vi "Core_[HSMS]Selected.vi"(8 "error in (no error)":errorcluster, 11 "HSMS Class in":refnum<class "HSMS Class.lvclass">) -> (0 "error out":errorcluster, 3 "HSMS Class out":refnum<class "HSMS Class.lvclass">)   [LabVIEW 2020, in "SECS Communication.lvlib" / "HSMS Class.lvclass"]
uses:
  HSMS Class.lvclass
  Notifier Type.ctl
  Message Packet.ctl
  Message Header.ctl
  PType.ctl
  SType.ctl
  HSMS State.ctl
  HSMS Class.lvclass/HSMS Class.ctl
  S9 Message Class/S9 Message Class.lvclass
  D:/Dropbox/SECS/SECS_GEM v1.1.2/Com/SECS Communication/SECS-II Class/SECS-II Class.lvclass
  Command Data.ctl
  SECS-II Class/SECS-II Class.lvclass
  Read Session ID.vi
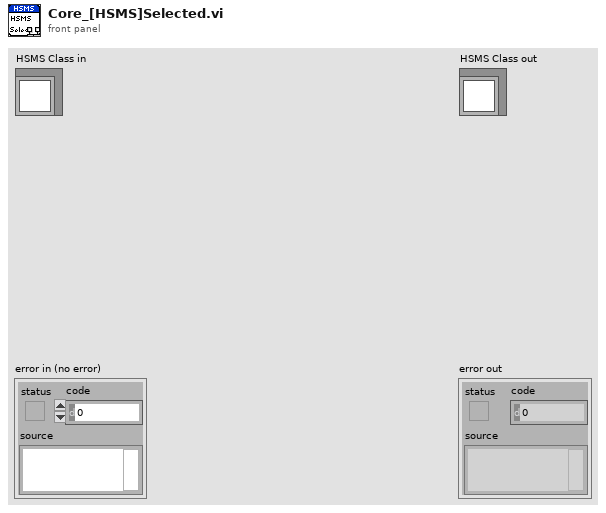
[diagram p1: front panel]
types:
  T1 = typedef "SECS Communication.lvlib/HSMS Class.lvclass/Message Packet.ctl" = cluster{"Message Header Cluster":T2, "Message Header":u8[], "Message Text":u8[]}
  T2 = typedef "SECS Communication.lvlib/HSMS Class.lvclass/Message Header.ctl" = cluster{"Byte 0-1(Session ID)":u16, "W-Bit":bool, "Byte 2":u8, "Byte 3":u8, "Byte 4(PType)":T3, "Byte 5(SType)":T4, "Byte 6-9(System Btyes)":u8[]}
  T3 = typedef "SECS Communication.lvlib/HSMS Class.lvclass/PType.ctl" = enum8{"SECS-II Encoding", "Reserved"}
  T4 = typedef "SECS Communication.lvlib/HSMS Class.lvclass/SType.ctl" = enum8{"Data Message", "Select.req", "Select.rsp", "Deselect.req", "Deselect.rsp", "Linktest.req", "Linktest.rsp", "Reject.req", "Separate.req"}
  T5 = typedef "SECS Communication.lvlib/HSMS Class.lvclass/Notifier Type.ctl" = enum16{"TCPIP Connect", "TCPIP Disconnect", "Receive Message", "Send Message", "T3 Timeout", "T6 Timeout", "T7 Timeout", "Error", "Stop"}
  T6 = typedef "SECS Communication.lvlib/HSMS Class.lvclass/HSMS State.ctl" = enum16{"[TCP/IP]Not Connect", "[HSMS]Not Selected", "[HSMS]Selected", "Stop"}
  T7 = typedef "SECS Communication.lvlib/HSMS Class.lvclass/Command Data.ctl" = cluster{"SECS-II Class":refnum<class "SECS-II Class.lvclass">, "Reply Notifier":refnum<notifier>}
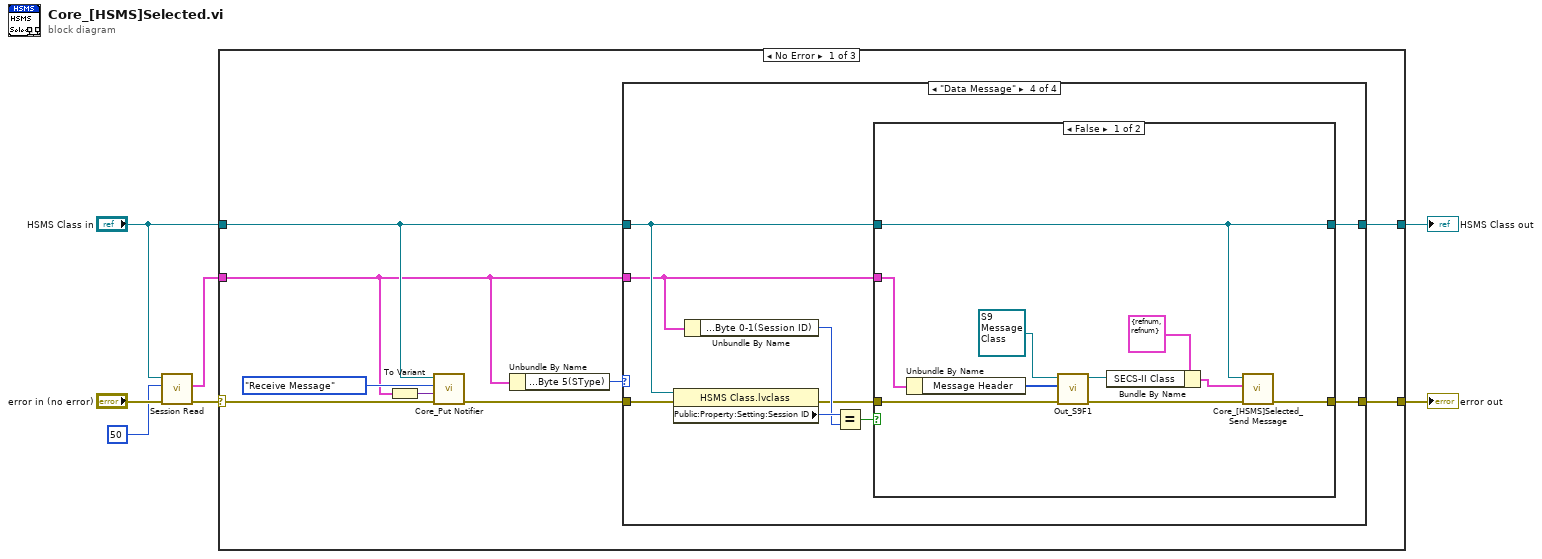
[diagram p0: block diagram]
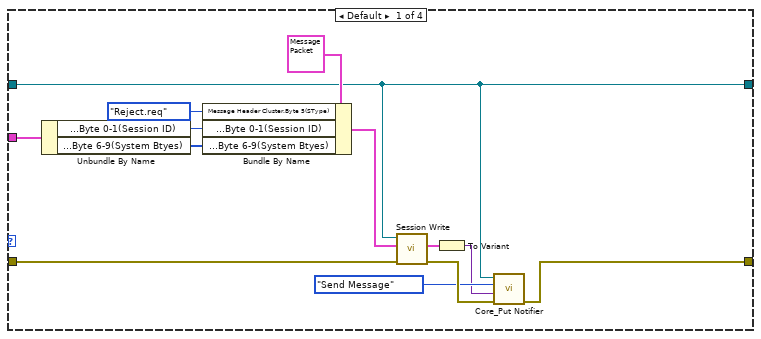
[diagram p2: hidden frame]
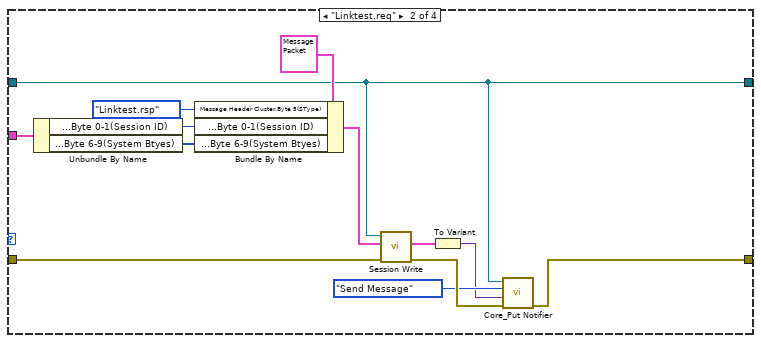
[diagram p3: hidden frame]
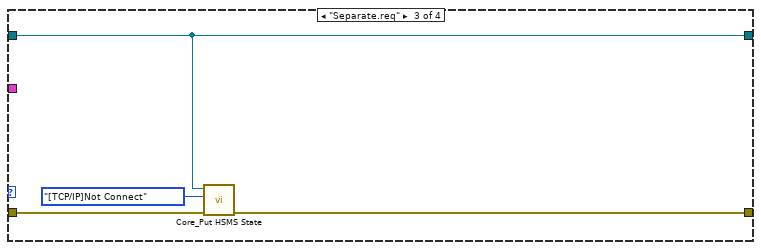
[diagram p4: hidden frame]
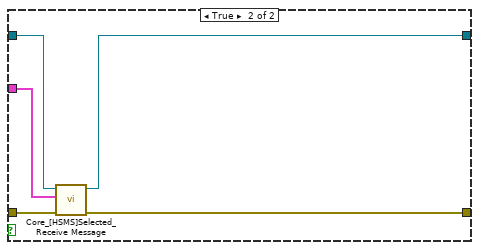
[diagram p5: hidden frame]
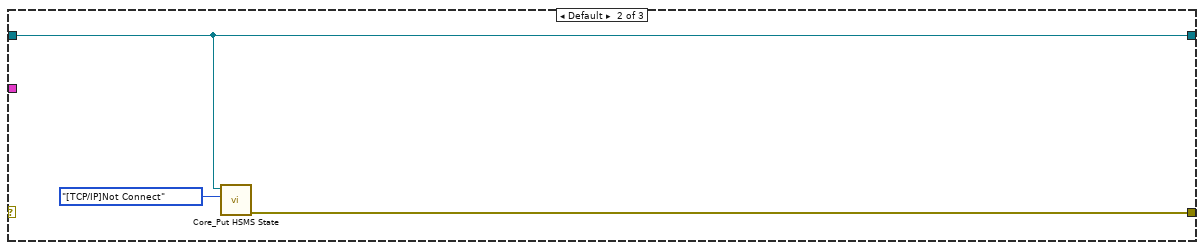
[diagram p6: hidden frame]
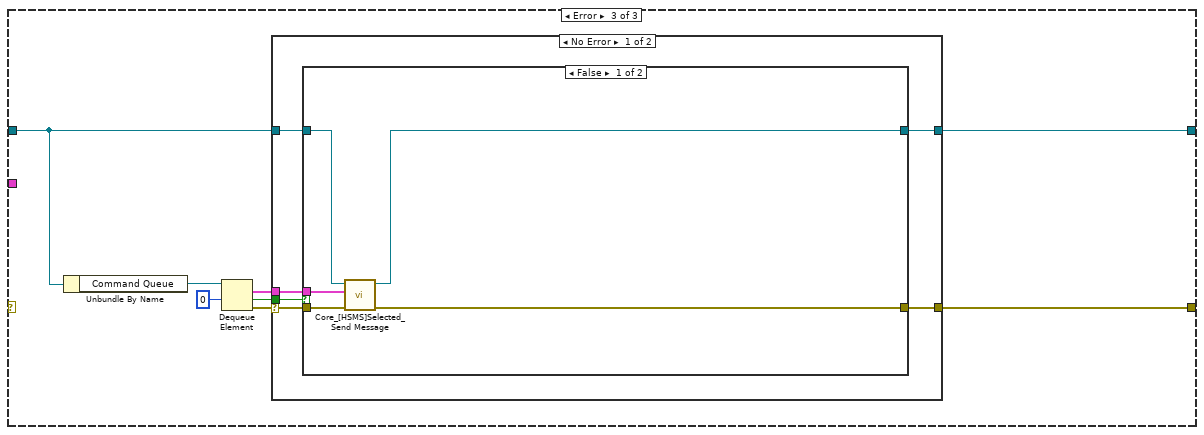
[diagram p7: hidden frame]
diagram:
  n1 = call "Session Read.vi"("error in (no error)"="error in (no error)", "Timeout"=50, "HSMS Class in"="HSMS Class in") -> ("error out"=w2:errorcluster, "Message Packet"=w1:T1)  [unwired: 6 in, 1 out]
  n2 = case shown="No Error" w2 {
    selector: w2 -> [w12 _ _]
    tunnel: "HSMS Class in" -> [w10 w72 w78]
    tunnel: w1 -> [w8 _ _]
    tunnel: [w16 w72 w77] -> w4
    tunnel: [w15 w73 w75] -> w3
    frame No Error {
      n3 = To Variant(anything=w8) -> (Variant=w13:variant)
      n4 = call "Core_Put Notifier.vi"("error in (no error)"=w12, "Data"=w13, "Notifier Type"=Notifier_Type."Receive Message", "HSMS Class in"=w10) -> ("error out"=w11:errorcluster)  [unwired: 6 in, 1 out]
      n5 = Unbundle By Name(w8) -> ("Message Header Cluster.Byte 5(SType)"=w9:T4)
      n6 = case shown="\"Data Message\"" w9 {
        tunnel: w10 -> [w21 w34 w45 w51]
        tunnel: [w21 w34 w45 w55] -> w16
        tunnel: w11 -> [w24 w37 w46 w52]
        tunnel: w8 -> [w29 w42 _ w50]
        tunnel: [w22 w35 w44 w54] -> w15
        frame Default {
          n7 = Unbundle By Name(w29) -> ("Message Header Cluster.Byte 0-1(Session ID)"=w27:u16, "Message Header Cluster.Byte 6-9(System Btyes)"=w25:u8[])
          n8 = Bundle By Name(cluster=T1 {"Message Header Cluster"={"Byte 0-1(Session ID)"=0, "W-Bit"=FALSE, "Byte 2"=0, "Byte 3"=0, "Byte 4(PType)"=enum."SECS-II Encoding", "Byte 5(SType)"=enum."Data Message", "Byte 6-9(System Btyes)"=[]}, "Message Header"=[], "Message Text"=[]} ("Message Packet"), "Message Header Cluster.Byte 5(SType)"=SType."Reject.req" ("Message Header.Byte 5(SType)"), "Message Header Cluster.Byte 0-1(Session ID)"=w27, "Message Header Cluster.Byte 6-9(System Btyes)"=w25) -> (w19:T1)
          n9 = call "Session Write.vi"("error in (no error)"=w24, "Message Packet In"=w19, "HSMS Class in"=w21) -> ("error out"=w23:errorcluster, "Message Packet Out"=w17:T1)  [unwired: 6 in, 1 out]
          n10 = To Variant(anything=w17) -> (Variant=w18:variant)
          n11 = call "Core_Put Notifier.vi"("error in (no error)"=w23, "Data"=w18, "Notifier Type"=Notifier_Type."Send Message", "HSMS Class in"=w21) -> ("error out"=w22:errorcluster)  [unwired: 6 in, 1 out]
        }
        frame "Linktest.req" {
          n12 = Unbundle By Name(w42) -> ("Message Header Cluster.Byte 0-1(Session ID)"=w40:u16, "Message Header Cluster.Byte 6-9(System Btyes)"=w38:u8[])
          n13 = Bundle By Name(cluster=T1 {"Message Header Cluster"={"Byte 0-1(Session ID)"=0, "W-Bit"=FALSE, "Byte 2"=0, "Byte 3"=0, "Byte 4(PType)"=enum."SECS-II Encoding", "Byte 5(SType)"=enum."Data Message", "Byte 6-9(System Btyes)"=[]}, "Message Header"=[], "Message Text"=[]} ("Message Packet"), "Message Header Cluster.Byte 5(SType)"=SType."Linktest.rsp" ("Message Header.Byte 5(SType)"), "Message Header Cluster.Byte 0-1(Session ID)"=w40, "Message Header Cluster.Byte 6-9(System Btyes)"=w38) -> (w32:T1)
          n14 = call "Session Write.vi"("error in (no error)"=w37, "Message Packet In"=w32, "HSMS Class in"=w34) -> ("error out"=w36:errorcluster, "Message Packet Out"=w30:T1)  [unwired: 6 in, 1 out]
          n15 = To Variant(anything=w30) -> (Variant=w31:variant)
          n16 = call "Core_Put Notifier.vi"("error in (no error)"=w36, "Data"=w31, "Notifier Type"=Notifier_Type."Send Message", "HSMS Class in"=w34) -> ("error out"=w35:errorcluster)  [unwired: 6 in, 1 out]
        }
        frame "Separate.req" {
          n17 = call "Core_Put HSMS State.vi"("error in (no error)"=w46, "HSMS State"=HSMS_State."[TCP/IP]Not Connect", "HSMS Class in"=w45) -> ("error out"=w44:errorcluster)  [unwired: 7 in, 1 out]
        }
        frame "Data Message" {
          n18 = property class="HSMS Class.lvclass"(reference=w51, error in=w52) -> (error out=w48:errorcluster, "Public:Property:Setting:Session ID"=w53:u16)  [unwired: 1 out]
          n19 = Unbundle By Name(w50) -> ("Message Header Cluster.Byte 0-1(Session ID)"=w49:u16)
          n20 = Equal?(x=w53, y=w49) -> (x = y?=w47:bool)
          n21 = case shown="False" w47 {
            tunnel: [w58 w70] -> w55
            tunnel: [w59 w69] -> w54
            tunnel: w51 -> [w58 w68]
            tunnel: w50 -> [w57 w67]
            tunnel: w48 -> [w60 w66]
            frame False {
              n22 = Unbundle By Name(w57) -> ("Message Header"=w56:u8[])
              n23 = call "Out_S9F1.vi"("error in (no error)"=w60, "Message Header"=w56, "S9 Message Class in"=refnum<class "S9 Message Class.lvclass"> refnum) -> ("error out"=w63:errorcluster, "S9 Message Class out"=w64:refnum<class "S9 Message Class.lvclass">)  [unwired: 7 in]
              n24 = Bundle By Name(cluster=T7 {"SECS-II Class"=refnum, "Reply Notifier"=refnum} ("Command Data"), "SECS-II Class"=w64) -> (w65:T7)
              n25 = call "Core_[HSMS]Selected_Send Message.vi"("error in (no error)"=w63, "Command Data"=w65, "HSMS Class in"=w58) -> ("error out"=w59:errorcluster)  [unwired: 7 in, 1 out]
            }
            frame True {
              n26 = call "Core_[HSMS]Selected_Receive Message.vi"("error in (no error)"=w66, "Message Packet"=w67, "HSMS Class in"=w68) -> ("error out"=w69:errorcluster, "HSMS Class out"=w70:refnum<class "HSMS Class.lvclass">)  [unwired: 7 in]
            }
          }
        }
      }
    }
    frame Default {
      n27 = call "Core_Put HSMS State.vi"("HSMS State"=HSMS_State."[TCP/IP]Not Connect", "HSMS Class in"=w72) -> ("error out"=w73:errorcluster)  [unwired: 8 in, 1 out]
    }
    frame Error {
      n28 = Unbundle By Name(w78) -> ("Command Queue"=w81:refnum<queue>)
      n29 = Dequeue Element(queue=w81, timeout in ms (-1)=0) -> (element=w74:T7, timed out?=w76:bool, error out=w79:errorcluster)  [unwired: 1 in, 1 out]
      n30 = case shown="No Error" w79 {
        selector: w79 -> [w86 _]
        tunnel: w78 -> [w84 w95]
        tunnel: [w83 w95] -> w77
        tunnel: w76 -> [w87 _]
        tunnel: [w85 _] -> w75
        tunnel: w74 -> [w82 _]
        frame No Error {
          n31 = case shown="False" w87 {
            tunnel: w86 -> [w92 w93]
            tunnel: [w89 w93] -> w85
            tunnel: w84 -> [w91 w94]
            tunnel: [w90 w94] -> w83
            tunnel: w82 -> [w88 _]
            frame False {
              n32 = call "Core_[HSMS]Selected_Send Message.vi"("error in (no error)"=w92, "Command Data"=w88, "HSMS Class in"=w91) -> ("error out"=w89:errorcluster, "HSMS Class out"=w90:refnum<class "HSMS Class.lvclass">)  [unwired: 7 in]
            }
            frame True {
              # "Timeout"
            }
          }
        }
        frame Error {
        }
      }
    }
  }
  "error out" <- w3
  "HSMS Class out" <- w4
